vi "SSL Detection Robot.vi"(5 "Time Stamp":timestamp, 8 "error in":errorcluster, 9 "Array":u8[](array[numeric]) format="%02x") -> (0 "error out":errorcluster, 1 "Length-delimited":u8[](array[numeric]) format="%02x", 3 "Detection Robot":T1)   [LabVIEW 2016]
uses:
  SSL Detection Robot.ctl
  Varint Decoder uint32.vi
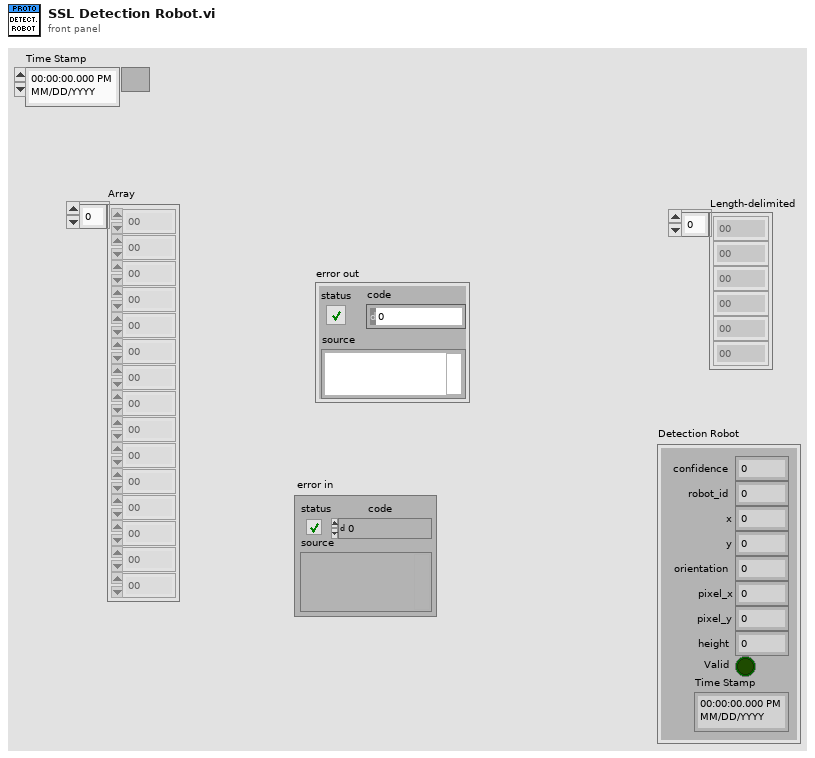
[diagram p1: front panel]
types:
  T1 = typedef "SSL Detection Robot.ctl" = cluster{"x":dbl, "robot_id":u32, "confidence":sgl, "y":sgl, "orientation":sgl, "pixel_x":sgl, "pixel_y":sgl, "height":sgl, "Valid":bool, "Time Stamp":timestamp}
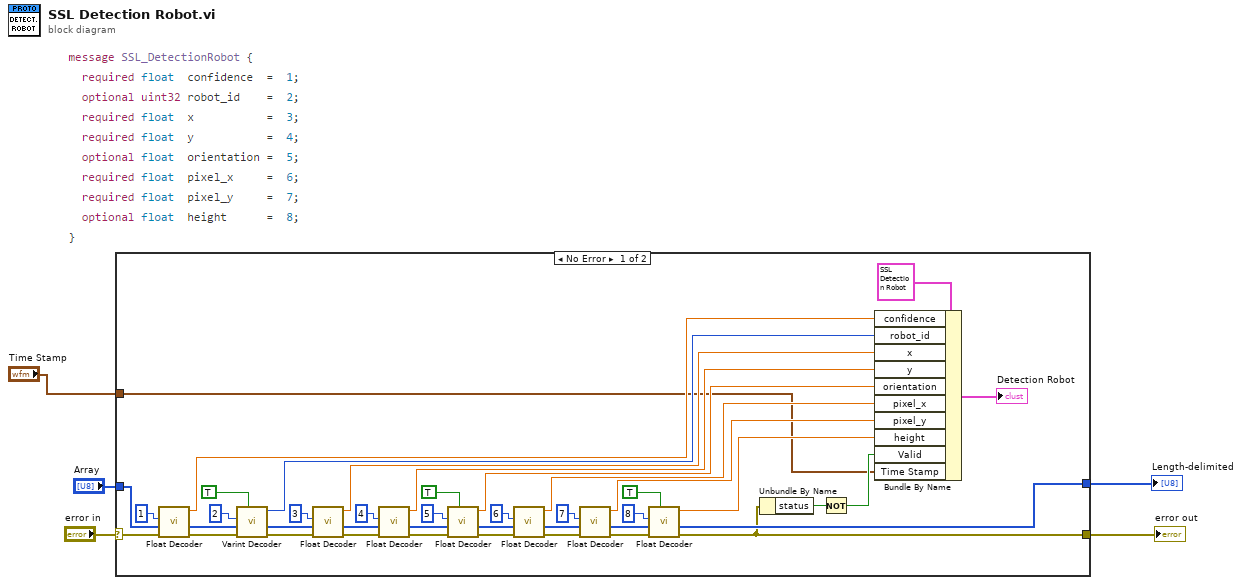
[diagram p0: block diagram]
diagram:
  n1 = case shown="No Error" "error in" {
    selector: "error in" -> [w46 w49]
    tunnel: [w9 w49] -> w4
    tunnel: [w24 w48] -> w3
    tunnel: "Array" -> [w12 w48]
    tunnel: "Time Stamp" -> [w6 _]
    frame No Error {
      n2 = call "Float Decoder.vi"("error in (no error)"=w46, "Array"=w12, "Key"=1) -> ("error out"=w45:errorcluster, "array w/ subset deleted"=w11:u8[], "Float"=w33:sgl)  [unwired: 5 in, 1 out]
      n3 = call-poly "Varint Decoder.vi"("Optional"=TRUE, "error in (no error)"=w45, "Array"=w11, "Key"=2) -> ("error out"=w44:errorcluster, "array w/ subset deleted"=w14:u8[], "Varint"=w32:u32)  [unwired: 4 in, 1 out]
      n4 = call "Float Decoder.vi"("error in (no error)"=w44, "Array"=w14, "Key"=3) -> ("error out"=w43:errorcluster, "array w/ subset deleted"=w15:u8[], "Float"=w31:sgl)  [unwired: 5 in, 1 out]
      n5 = call "Float Decoder.vi"("error in (no error)"=w43, "Array"=w15, "Key"=4) -> ("error out"=w38:errorcluster, "array w/ subset deleted"=w16:u8[], "Float"=w30:sgl)  [unwired: 5 in, 1 out]
      n6 = call "Float Decoder.vi"("Optional"=TRUE, "error in (no error)"=w38, "Array"=w16, "Key"=5) -> ("error out"=w36:errorcluster, "array w/ subset deleted"=w18:u8[], "Float"=w29:sgl)  [unwired: 4 in, 1 out]
      n7 = call "Float Decoder.vi"("error in (no error)"=w36, "Array"=w18, "Key"=6) -> ("error out"=w34:errorcluster, "array w/ subset deleted"=w19:u8[], "Float"=w28:sgl)  [unwired: 5 in, 1 out]
      n8 = call "Float Decoder.vi"("error in (no error)"=w34, "Array"=w19, "Key"=7) -> ("error out"=w26:errorcluster, "array w/ subset deleted"=w20:u8[], "Float"=w10:sgl)  [unwired: 5 in, 1 out]
      n9 = call "Float Decoder.vi"("Optional"=TRUE, "error in (no error)"=w26, "Array"=w20, "Key"=8) -> ("error out"=w9:errorcluster, "array w/ subset deleted"=w24:u8[], "Float"=w25:sgl)  [unwired: 4 in, 1 out]
      n10 = Unbundle By Name(w9) -> ("status"=w8:bool)
      n11 = Not(x=w8) -> (.not. x?=w7:bool)
      n12 = Bundle By Name(cluster=T1 {"x"=0.0, "robot_id"=0, "confidence"=0.0, "y"=0.0, "orientation"=0.0, "pixel_x"=0.0, "pixel_y"=0.0, "height"=0.0, "Valid"=FALSE, "Time Stamp"=timestamp(0 s since 1904-01-01)} ("Detection Robot 2"), "confidence"=w33, "robot_id"=w32, "x"=w31, "y"=w30, "orientation"=w29, "pixel_x"=w28, "pixel_y"=w10, "height"=w25, "Valid"=w7, "Time Stamp"=w6) -> (→"Detection Robot":T1)
    }
    frame Error {
    }
  }
  "error out" <- w4
  "Length-delimited" <- w3
